vi "File.Move File to New Folder.vi"(7 "Action":enum16{"Move", "Copy"}(ring), 8 "error in":errorcluster, 10 "Destination Folder":path, 11 "Source File Path":path) -> (0 "error out":errorcluster, 3 "New Path":path)   [LabVIEW 2018]
uses:
  Errors/Error.Error Code List.ctl
  <vilib>/KATE/Files/File Utils.lvlib
panel:
  out "Dir":bool
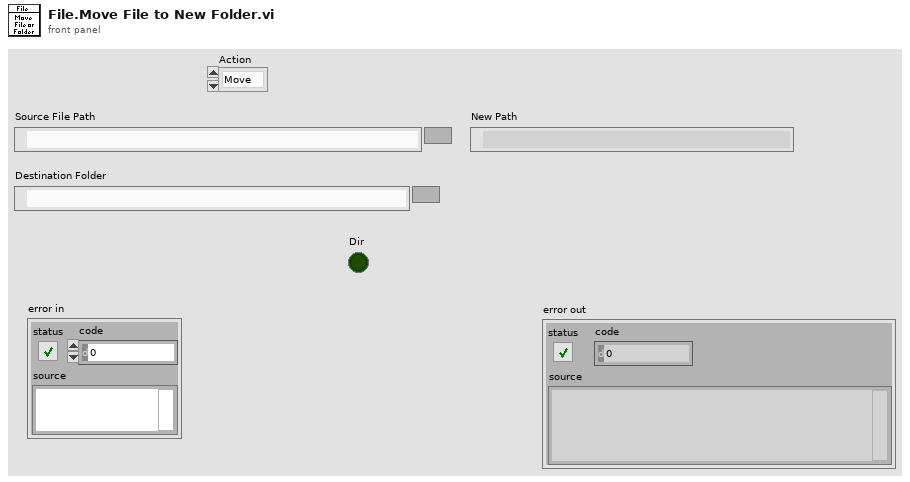
[diagram p1: front panel]
types:
  T1 = typedef "Error.Error Code List.ctl" = i32
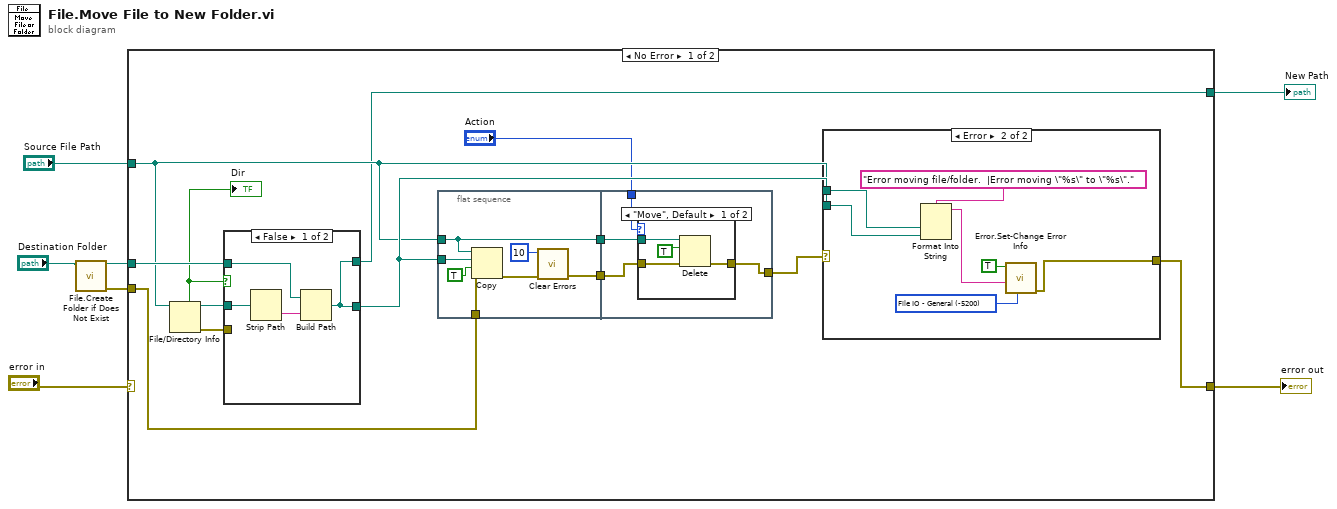
[diagram p0: block diagram]
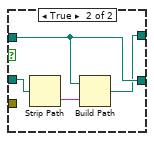
[diagram p2: hidden frame]
diagram:
  n1 = call <vilib>:"File.Create Folder if Does Not Exist.vi"("Path"="Destination Folder") -> ("error out"=w1:errorcluster, "Dup Path"=w3:path)  [unwired: 8 in, 1 out]
  n2 = case shown="No Error" "error in" {
    selector: "error in" -> [_ w52]
    tunnel: w3 -> [w20 _]
    tunnel: "Source File Path" -> [w14 _]
    tunnel: [w18 w52] -> w6
    tunnel: [w9 _] -> w5
    tunnel: w1 -> [w10 _]
    frame No Error {
      n3 = File/Directory Info(path=w14) -> (path out=w13:path, directory=w12:bool, error out=w11:errorcluster)  [unwired: 1 in, 4 out]
      "Dir" <- w12
      n4 = case shown="False" w12 {
        tunnel: w20 -> [w23 w26]
        tunnel: [w21 w26] -> w19
        tunnel: w13 -> [w22 w27]
        tunnel: w11 -> [_ _]
        tunnel: [w21 w25] -> w9
        frame False {
          n5 = Strip Path(path=w22) -> (name=w24:string)  [unwired: 1 out]
          n6 = Build Path(base path=w23, name or relative path=w24) -> (appended path=w21:path)
        }
        frame True {
          n7 = Strip Path(path=w27) -> (name=w28:string)  [unwired: 1 out]
          n8 = Build Path(base path=w26, name or relative path=w28) -> (appended path=w25:path)
        }
      }
      n9 = flat-sequence {
        tunnel: w14 -> [w34]
        tunnel: w19 -> [w35]
        tunnel: [w34] -> w17
        tunnel: [w33] -> w15
        tunnel: w10 -> [w29]
        tunnel: w17 -> [w39]
        tunnel: [w37] -> w16
        tunnel: w15 -> [w38]
        tunnel: "Action" -> [w36]
        frame #0 {
          n10 = Copy(8:w29, 9:TRUE ("overwrite (F)"), 10:w35, 11:w34) -> (0:w32:errorcluster)  [unwired: 1 in, 2 out]
          n11 = call <vilib>:"Clear Errors.vi"("error in (no error)"=w32, "specific error code to clear (0: all)"=10) -> ("error out"=w33:errorcluster)  [unwired: 4 in, 1 out]
        }
        frame #1 {
          n12 = case shown="\"Move\", Default" w36 {
            tunnel: w39 -> [w43 _]
            tunnel: w38 -> [w41 w44]
            tunnel: [w40 w44] -> w37
            frame "Move", Default {
              n13 = Delete(path (use dialog)=w43, entire hierarchy (F)=TRUE, error in=w41) -> (error out=w40:errorcluster)  [unwired: 2 in, 2 out]
            }
            frame "Copy" {
            }
          }
        }
      }
      n14 = case shown="Error" w16 {
        tunnel: w14 -> [_ w51]
        tunnel: w19 -> [_ w50]
        tunnel: [_ w45] -> w18
        frame No Error {
        }
        frame Error {
          w47 = T1 -5200 items=["No Error"=0, "Abort"=-2, "Misc"=-5000, "Fixture Error"=-5100, "File IO - General"=-5200, "FIle IO - Config Error"=-5201, "Instrument - General"=-5300, "Instrument - Serial Com"=-5301, "Instrument - Camera"=-5302, "Instrument - PS"=-5303, "Instrument - Oscilloscope"=-5304, "Instrument - Function Gen"=-5305, "Instrument - Load"=-5306, "Instrument - Meter"=-5307, "Instrument - Power Control"=-5308, "Instrument - Motion"=-5309, "Instrument - RF"=-5310, "System Exe"=-5400, "Image Processing"=-5500, "Communication"=-5600, "Script - Syntax Error"=-6000, "Script - Invalid Name or Param"=-6100, "Script - Timeout"=-6200, "Invalid Data"=-6300, "FW Update Error"=-6500] ("Std Code")
          n15 = Format Into String(format string="Error moving file/folder.  |Error moving \"%s\" to \"%s\".", w51, w50) -> (resulting string=w46:string)  [unwired: 2 in, 1 out]
          n16 = call "Error.Set-Change Error Info.vi"("Std Code"=w47, "Description"=w46, "Set Error"=TRUE) -> ("error out"=w45:errorcluster)  [unwired: 8 in]
        }
      }
    }
    frame Error {
    }
  }
  "New Path" <- w5
  "error out" <- w6
